vi "Setstring_value.vi"(8 "error in (no error)":errorcluster, 10 "Set_Val":string, 11 "OneOfTemplate in":refnum<class "ni_protobuf_types_WaveformAttributeValue_attribute.lvclass">) -> (0 "error out":errorcluster, 3 "OneOfTemplate out":refnum<class "ni_protobuf_types_WaveformAttributeValue_attribute.lvclass">)   [LabVIEW 2020, in "ni.protobuf.types.lvlib" / "ni_protobuf_types_WaveformAttributeValue_attribute.lvclass"]
uses:
  ni_protobuf_types_WaveformAttributeValue_attribute.lvclass
  ni_protobuf_types_WaveformAttributeValue_attribute.lvclass/ni_protobuf_types_WaveformAttributeValue_attribute.ctl
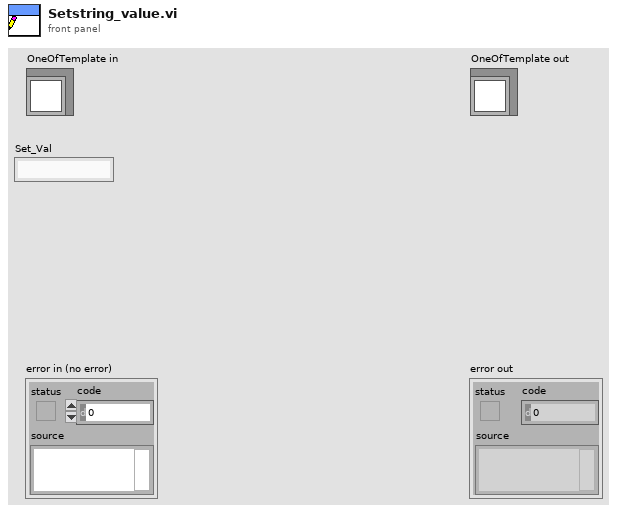
[diagram p1: front panel]
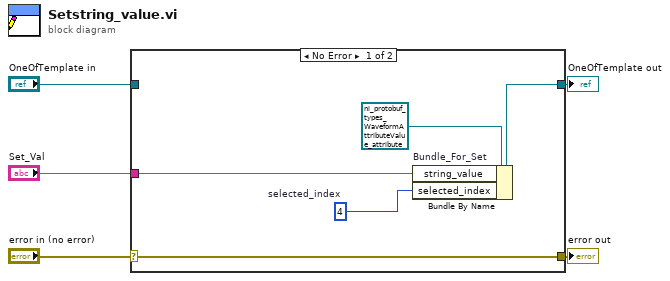
[diagram p0: block diagram]
diagram:
  n1 = case shown="No Error" "error in (no error)" {
    selector: "error in (no error)" -> [w10 w11]
    tunnel: [w10 w11] -> w4
    tunnel: [w9 w12] -> w2
    tunnel: "OneOfTemplate in" -> [_ w12]
    tunnel: "Set_Val" -> [w8 _]
    frame No Error {
      w7 = 4  # selected_index
      n2 = Bundle By Name "Bundle_For_Set"(cluster=refnum<class "ni_protobuf_types_WaveformAttributeValue_attribute.lvclass"> refnum ("OneOfTemplate in"), "string_value"=w8, "selected_index"=w7) -> (w9:refnum<class "ni_protobuf_types_WaveformAttributeValue_attribute.lvclass">)
    }
    frame Error {
    }
  }
  "error out" <- w4
  "OneOfTemplate out" <- w2
